vi "filter.post.state.vi"(11 "filter.data in":T1 {"memory.command"."order.slot.value"."Quantity" format="%016x"; "memory.command"."order.slot.value"."OrderId" format="%016x"; "memory.command"."ticker.slot.value"."Symbol" format="%016x"; "Scratch"."OrderId" format="%016x"}) -> (3 "filter.data out 2":T1 {"memory.command"."order.slot.value"."Quantity" format="%016x"; "memory.command"."order.slot.value"."OrderId" format="%016x"; "memory.command"."ticker.slot.value"."Symbol" format="%016x"; "Scratch"."OrderId" format="%016x"})   [LabVIEW 2020]
uses:
  filter.data.ctl
  filter.states.ctl
  filter.debug.ctl
  filter.debug.slot.ctl
  filter.data.scratch.ctl
  builds/fpganow.common/orderbook.command.ctl
  builds/fpganow.common/orderbook.command.type.ctl
  filter.memory.command.ctl
  ticker.slot.ctl
  order.slot.ctl
  filter.getstate.ctl
  filter.getstate.slot.ctl
  <vilib>/rvi/DataTransferAndStorage/Container/Common/niFpgaContainerGetUniqueNameForEmu.vi
  <vilib>/rvi/DataTransferAndStorage/Container/Common/niFpgaContainerSetEmuInfo.vi
  <vilib>/rvi/eio/common/nirviEmuReportErrorAndStop.vi
  <vilib>/rvi/Emulation/niFpgaEmulationIsFPGAContextNoSignature.vi
  <vilib>/rvi/Emulation/niFpgaSctlEmulationGetInTimedLoop.vi
  <vilib>/rvi/errors/niFpgaSetErrorForExecOnDevCompSimple.vi
  <vilib>/rvi/FIFO/Fifo_Resource/nirvififoEmulationSetSize.vi
  <vilib>/rvi/FIFO/Fifo_Resource/nirviFifoEmulationQueueMgr.vi
  <instcachedir>/0/nirviFifoEmulationQueueMgr_E5CAEC123FF24DC58D834DCA3CDAA9B5.lvgen/nirviFifoEmulationQueueMgr_E5CAEC123FF24DC58D834DCA3CDAA9B5_008.vi
  <vilib>/rvi/FIFO/Fifo_Resource/nirvififoEmulationDetermineInputValidOut.vi
  <vilib>/rvi/FIFO/Fifo_Resource/nirvififoEmulationCreateLock.vi
  <vilib>/rvi/Emulation/niFpgaProcessEmulError.vi
  <vilib>/rvi/FIFO/Fifo_Resource/nirvififoEmulationObtainLock.vi
  <vilib>/rvi/FIFO/Fifo_Resource/nirvififoEmulationReleaseLock.vi
  <vilib>/rvi/occurrence/nirviWaitOnOccurrenceBase.vi
  <vilib>/rvi/errors/nirviReportUnexpectedCaseInternalError.vi
  <vilib>/rvi/errors/nirviReportUnexpectedCaseInternalError (U32).vi
  <instcachedir>/0/nirviFifoEmulationQueueMgr_E5CAEC123FF24DC58D834DCA3CDAA9B5.lvgen/nirviFifoEmulationQueueMgr_E5CAEC123FF24DC58D834DCA3CDAA9B5_013.vi
  <vilib>/rvi/DataTransferAndStorage/Container/Common/niFpgaContainerExecOnDevCompGetState.vi
  <vilib>/rvi/Memory/Memory_Emulation/niFpgaMemoryEmulationCacheClearOnFirstRun.vi
  <vilib>/rvi/Memory/Memory_Emulation/nirvimemoryEmulationManagerCache_MakeExclusive.vi
  <vilib>/rvi/Memory/Memory_Emulation/niFpgaMemoryEmulationValidateCache.vi
  <vilib>/rvi/Memory/Memory_Emulation/nirvimemoryEmulationManagerCache_InsertValue.vi
  <vilib>/Utility/error.llb/Clear Errors.vi
  <vilib>/rvi/Memory/Memory_Emulation/nirvimemoryEmulationManagerCache_ReleaseExclusive.vi
  <vilib>/rvi/Memory/Memory_Emulation/nirvimemoryEmulationManagerCache_GetValue.vi
  <vilib>/rvi/Memory/Memory_Emulation/nirvimemoryEmulationManagerCache_SetValue.vi
  <vilib>/rvi/Emulation/niFpgaSctlEmulationResourceMgr.vi
  <vilib>/rvi/LocalResourceManager/LocalResourceManager.xnode
  <vilib>/rvi/DataTransferAndStorage/Container/XNode/niFpgaContainer.xnode
  <vilib>/rvi/FIFO/Fifo_Resource/nirvififoEmulationWrite.vi
  <vilib>/rvi/Memory/Memory_Emulation/niFpgaMemoryEmulationRefIn.vi
  builds/fpganow.common/fpganow.common.fpga.lvlib
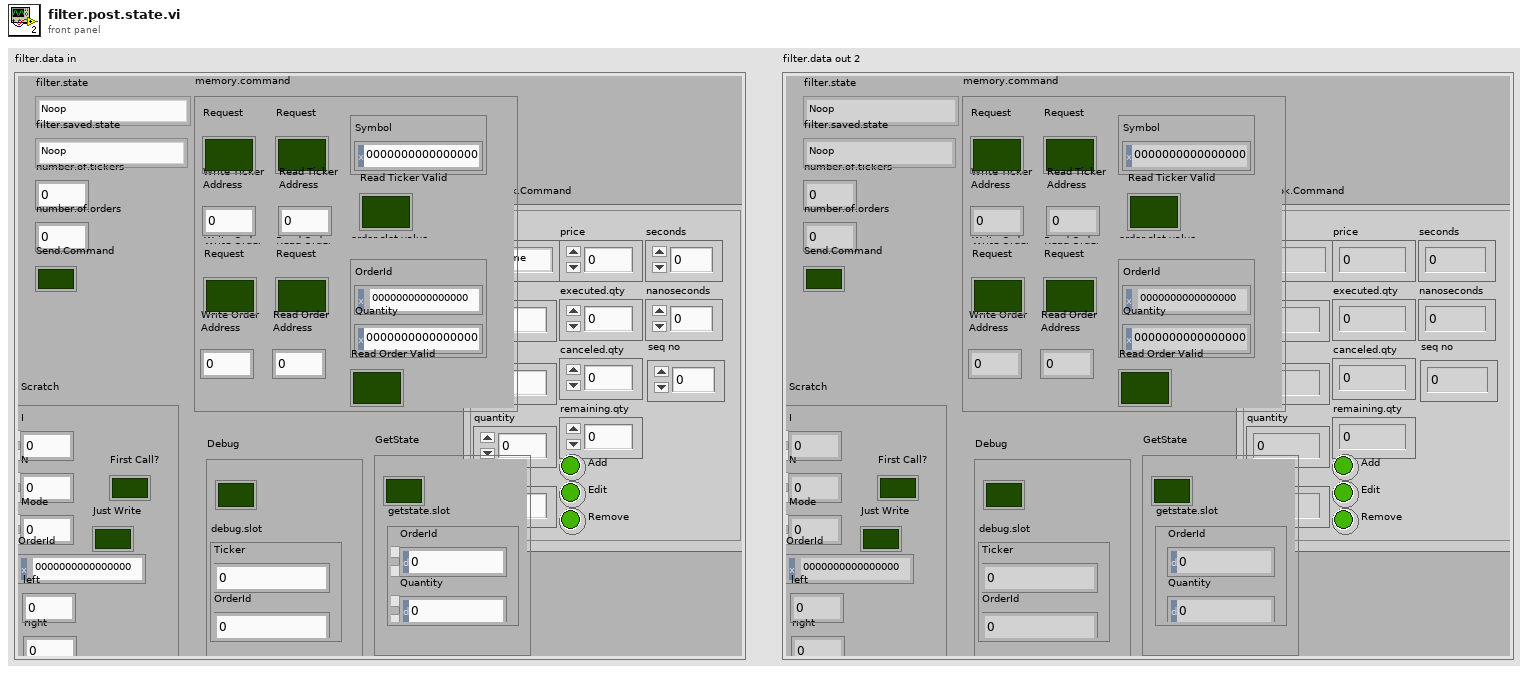
[diagram p1: front panel]
types:
  T1 = typedef "filter.data.ctl" = cluster{"filter.state":T2, "Debug":T3, "number.of.tickers":u32, "number.of.orders":u32, "filter.saved.state":T2, "Scratch":T5, "OrderBook.Command":T6, "Send.Command":bool, "memory.command":T8, "GetState":T11}
  T2 = typedef "filter.states.ctl" = enum16{"Noop", "Reset", "Debug", "Configuration", "Get.State", "Wait.for.Command", "Filter.Add", "Filter.Other", "Insert.Order", "Delete Order"}
  T3 = typedef "filter.debug.ctl" = cluster{"Write.to.Debug":bool, "debug.slot":T4}
  T4 = typedef "filter.debug.slot.ctl" = cluster{"Ticker":u64, "OrderId":u64}
  T5 = typedef "filter.data.scratch.ctl" = cluster{"I":u32, "N":u32, "Mode":u32, "OrderId":u64, "First Call?":bool, "Just Write":bool, "left":u32, "right":u32}
  T6 = typedef "fpganow.common.fpga.lvlib/orderbook.command.ctl" = cluster{"type":T7, "side":u8, "orderId ":u64, "quantity":u32, "symbol":u64, "price":u64, "executed.qty":u32, "canceled.qty":u32, "remaining.qty":u32, "seconds":u64, "nanoseconds":u64, "Add":bool, "Edit":bool, "Remove":bool, "seq no":u32}
  T7 = typedef "fpganow.common.fpga.lvlib/orderbook.command.type.ctl" = enum8{"Time", "AddOrder", "OrderExecuted", "OrderExecutedAtPrice", "ReduceSize", "ModifyOrder", "DeleteOrder", "Get.Everything", "Get.All.Orders", "Get.Top"}
  T8 = typedef "filter.memory.command.ctl" = cluster{"ticker.slot.value":T9, "order.slot.value":T10, "Write Ticker\nAddress":u32, "Write Ticker\nRequest":bool, "Read Ticker\nRequest":bool, "Read Ticker\nAddress":u32, "Read Ticker Valid":bool, "Write Order\nAddress":u32, "Write Order\nRequest":bool, "Read Order\nRequest":bool, "Read Order\nAddress":u32, "Read Order Valid":bool}
  T9 = typedef "ticker.slot.ctl" = cluster{"Symbol":u64}
  T10 = typedef "order.slot.ctl" = cluster{"OrderId":u64, "Quantity":u64}
  T11 = typedef "filter.getstate.ctl" = cluster{"Write.to.GetState":bool, "getstate.slot":T12}
  T12 = typedef "filter.getstate.slot.ctl" = cluster{"OrderId":u64, "Quantity":u64}
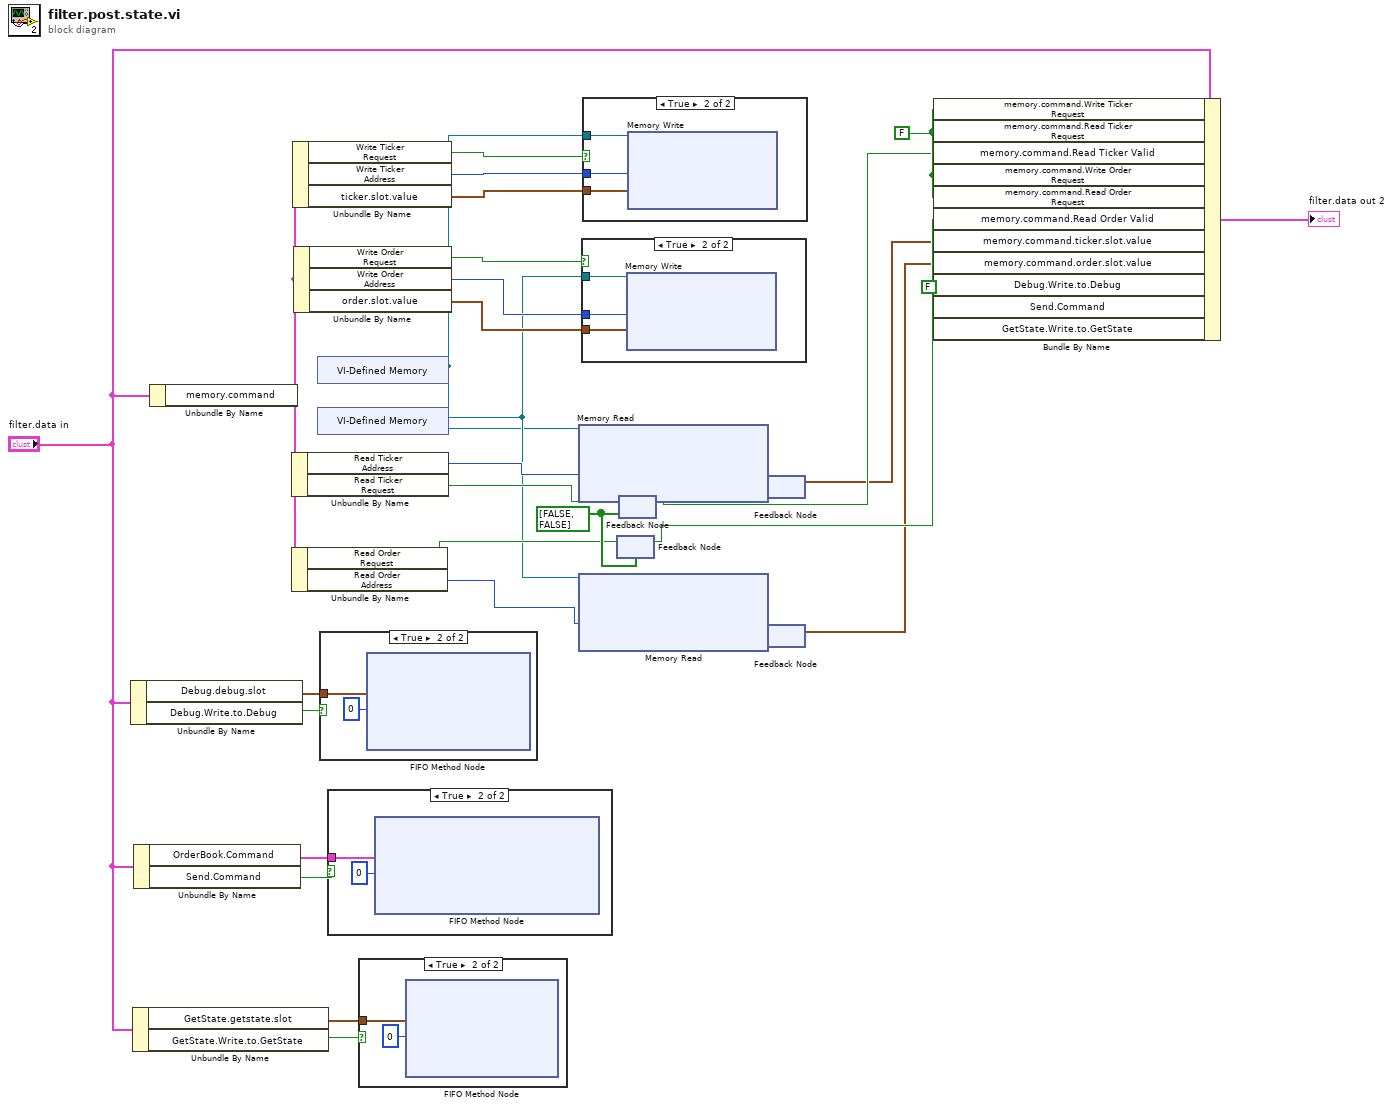
[diagram p0: block diagram]
diagram:
  w30 = FALSE ("memory.command.Write Ticker\nRequest")
  w27 = bool[] [FALSE, FALSE]
  w1 = FALSE ("Debug.Write.to.Debug")
  n1 = Unbundle By Name("filter.data in") -> ("Debug.debug.slot"=w15:T4, "Debug.Write.to.Debug"=w13:bool)
  n2 = Unbundle By Name("filter.data in") -> ("GetState.getstate.slot"=w2:T12, "GetState.Write.to.GetState"=w3:bool)
  n3 = Unbundle By Name("filter.data in") -> ("OrderBook.Command"=w17:T6, "Send.Command"=w16:bool)
  n4 = Unbundle By Name("filter.data in") -> ("memory.command"=w24:T8)
  n5 = Unbundle By Name(w24) -> ("Read Ticker\nAddress"=w8:u32, "Read Ticker\nRequest"=w23:bool)
  n6 = Unbundle By Name(w24) -> ("Read Order\nRequest"=w26:bool, "Read Order\nAddress"=w25:u32)
  n7 = Unbundle By Name(w24) -> ("Write Ticker\nRequest"=w18:bool, "Write Ticker\nAddress"=w5:u32, "ticker.slot.value"=w19:T9)
  n8 = Unbundle By Name(w24) -> ("Write Order\nRequest"=w20:bool, "Write Order\nAddress"=w21:u32, "order.slot.value"=w22:T10)
  n9 = xnode "VI-Defined Memory"() -> ("Memory Out"=w6:refnum<k21>)
  n10 = xnode "VI-Defined Memory"() -> ("Memory Out"=w7:refnum<k21>)
  n11 = case shown="True" w13 {
    tunnel: w15 -> [_ w32]
    frame False {
    }
    frame True {
      n12 = xnode ("FIFO Method Node")("Element"=w32, "Timeout"=0) -> ()  [unwired: 1 in, 2 out]
    }
  }
  n13 = case shown="True" w16 {
    tunnel: w17 -> [_ w33]
    frame False {
    }
    frame True {
      n14 = xnode ("FIFO Method Node")("Element"=w33, "Timeout"=0) -> ()  [unwired: 1 in, 2 out]
    }
  }
  n15 = case shown="True" w3 {
    tunnel: w2 -> [_ w36]
    frame False {
    }
    frame True {
      n16 = xnode ("FIFO Method Node")("Element"=w36, "Timeout"=0) -> ()  [unwired: 1 in, 2 out]
    }
  }
  n17 = xnode "Memory Read"("Address"=w8, "Memory In"=w6) -> ("Data"=w10:cluster{"Symbol":u64})  [unwired: 1 out]
  n18 = xnode "Memory Read"("Address"=w25, "Memory In"=w7) -> ("Data"=w9:cluster{"OrderId":u64, "Quantity":u64})  [unwired: 1 out]
  n19 = case shown="True" w20 {
    tunnel: w7 -> [_ w39]
    tunnel: w21 -> [_ w38]
    tunnel: w22 -> [_ w37]
    frame False {
    }
    frame True {
      n20 = xnode "Memory Write"("Address"=w38, "Data"=w37, "Memory In"=w39) -> ()  [unwired: 1 out]
    }
  }
  n21 = case shown="True" w18 {
    tunnel: w6 -> [_ w42]
    tunnel: w5 -> [_ w41]
    tunnel: w19 -> [_ w40]
    frame False {
    }
    frame True {
      n22 = xnode "Memory Write"("Address"=w41, "Data"=w40, "Memory In"=w42) -> ()  [unwired: 1 out]
    }
  }
  n23 = feedback #1(w27) -> (w29:bool)
  n24 = feedback-in #1(w26) -> ()
  n25 = feedback #2(w27) -> (w28:bool)
  n26 = feedback-in #2(w23) -> ()
  n27 = feedback #3() -> (w14:cluster{"Symbol":u64})  [unwired: 1 in]
  n28 = feedback-in #3(w10) -> ()
  n29 = feedback #4() -> (w12:cluster{"OrderId":u64, "Quantity":u64})  [unwired: 1 in]
  n30 = feedback-in #4(w9) -> ()
  n31 = Bundle By Name(cluster="filter.data in", "memory.command.Write Ticker\nRequest"=w30, "memory.command.Read Ticker\nRequest"=w30, "memory.command.Read Ticker Valid"=w28, "memory.command.Write Order\nRequest"=w30, "memory.command.Read Order\nRequest"=w30, "memory.command.Read Order Valid"=w29, "memory.command.ticker.slot.value"=w14, "memory.command.order.slot.value"=w12, "Debug.Write.to.Debug"=w1, "Send.Command"=w1, "GetState.Write.to.GetState"=w1) -> (→"filter.data out 2":T1)
